vi "Pop.vi"(0 "nb idice nv3":dbl) -> ()   [LabVIEW 2022 SP3]
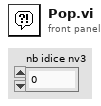
[diagram p1: front panel]
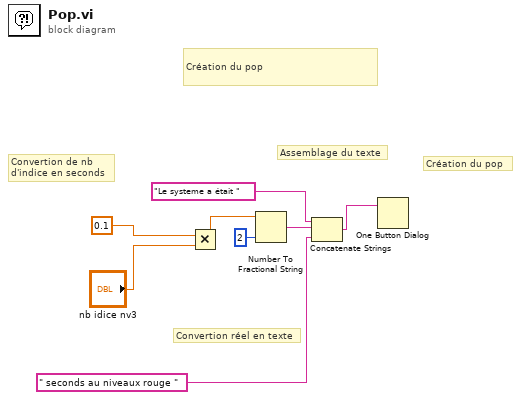
[diagram p0: block diagram]
diagram:
  # "Convertion de nb \nd'indice en seconds"
  # "Création du pop"
  # "Création du pop"
  # "Assemblage du texte"
  # "Convertion réel en texte"
  n1 = Multiply(x=0.1, y="nb idice nv3") -> (x*y=w3:dbl)
  n2 = Number To Fractional String(number=w3, precision (6)=i16 2) -> (F-format string=w6:string)  [unwired: 2 in]
  n3 = Concatenate Strings("Le systeme a était ", w6, " seconds au niveaux rouge " ("string")) -> (w4:string)
  n4 = One Button Dialog(message=w4) -> ()  [unwired: 1 in, 1 out]
